vi "EtaTransformation.vi"   [LabVIEW 2011]
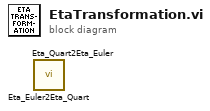
[diagram p0: block diagram]
diagram:
  n1 = call "Eta_Euler2Eta_Quart.vi"() -> ()  [unwired: 1 in, 1 out]
  n2 = call "Eta_Quart2Eta_Euler.vi"() -> ()  [unwired: 1 in, 1 out]
